vi "Periodic Tasks.vi"(8 "error in":errorcluster, 10 "Camera Occurance":refnum<k4>) -> ()   [LabVIEW 2017]
doc: "This VI runs in parallel to other tasks. It can contain as many user-defined periodic loops as you need. These can carry out PID or other sorts of timed response."
uses:
  <vilib>/Rock Robotics/WPI/ThirdParty/Sensors/navX/_TypeDefs/FRIC_navX_DeviceNumbersTypeDef.ctl
  <vilib>/Rock Robotics/WPI/ThirdParty/Sensors/navX/_Processing Loop/FRIC_navX_Internal_SPI_ProcessingLoop.vi
  _SHARE ALL/RoboRio Share All/Systems Share All/Joystick/Joystick.lvlib
  _SHARE ALL/RoboRio Share All/Systems Share All/System_Monitoring/System_Status.lvlib
  Systems/WCDrive2018/WCDrive2018.lvlib
  Systems/VisionHW Folder/VisionHW.lvlib
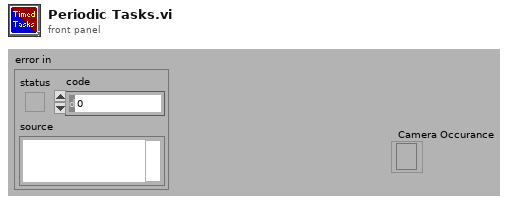
[diagram p1: front panel]
types:
  T1 = typedef "FRIC_navX_DeviceNumbersTypeDef.ctl" = enum16{"Dev0", "Dev1", "Dev2", "Dev3"}
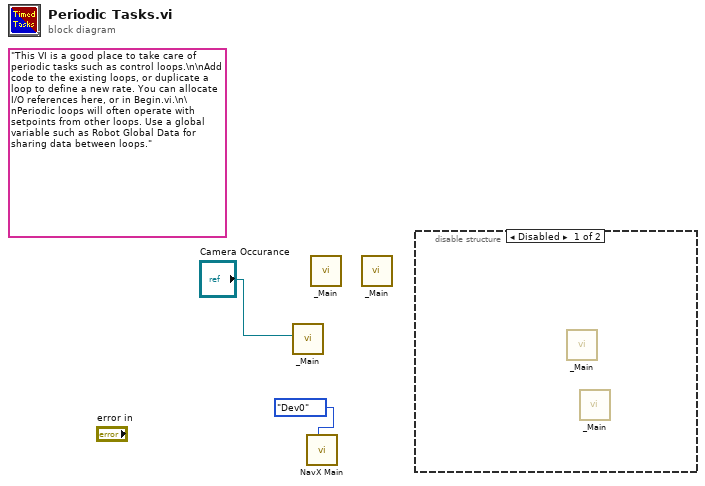
[diagram p0: block diagram]
diagram:
  (unwired) "This VI is a good place to take care of periodic tasks such as control loops.\n\nAdd code to the existing loops, or duplicate a loop to define a new rate. You can allocate I/O references here, or in Begin.vi.\n\nPeriodic loops will often operate with setpoints from other loops. Use a global variable such as Robot Global Data for sharing data between loops."
  n1 = call "_Main.vi"("Camera Occurance"="Camera Occurance") -> ()  [unwired: 11 in]
  n2 = call-poly <vilib>:"NavX Main.vi"("Device Number"=FRIC_navX_DeviceNumbersTypeDef."Dev0") -> ()  [unwired: 11 in]
  n3 = call "_Main.vi"() -> ()  [unwired: 12 in]
  n4 = call "_Main.vi"() -> ()  [unwired: 12 in]
  n5 = disable-structure shown="Disabled" {
    frame Disabled {
      n6 = call "_Main.vi"() -> ()  [unwired: 12 in]
      n7 = call "_Main.vi"() -> ()  [unwired: 12 in]
    }
    frame Enabled {
    }
  }
